vi "build-json-with-key.vi"(10 "value":variant, 11 "key":string) -> (3 "<JSON>First JSON Value\n\n<JSON>":string caption="<JSON>First JSON Value")   [LabVIEW 2019]
uses:
  1bc642b9-0734-4de5-ba9a-a56035824cc7.vi
  <vilib>/JDP Science/JSONtext/Variant to JSON Text.vi
  <vilib>/JDP Science/JSONtext/JSONtext.lvlib
panel:
  out "连接的字符串":string
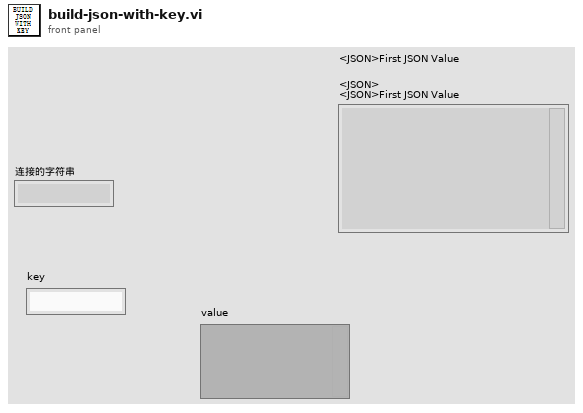
[diagram p1: front panel]
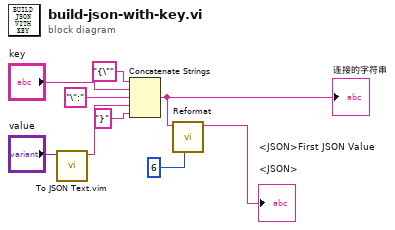
[diagram p0: block diagram]
diagram:
  n1 = call "To JSON Text.vim"("Anything"="value") -> ("<JSON>"=w6:string)  [unwired: 9 in, 1 out]
  n2 = Concatenate Strings("{\"" ("字符串"), "key", "\":" ("字符串"), w6, "}" ("字符串")) -> (w3:string)
  "连接的字符串" <- w3
  n3 = call <vilib>:"Reformat.vi"("Pretty Print Levels"=6, "JSON"=w3) -> ("<JSON>First JSON Value\n\n<JSON>"=→"<JSON>First JSON Value\n\n<JSON>":string)  [unwired: 6 in, 3 out]
